vi "1A Helper - Init Sensor.vi"(8 "error in (no error)":errorcluster, 11 "VISA Refnum in":refnum<visa-resource-name>="COM1") -> (0 "error out":errorcluster, 3 "VISA Refnum out":refnum<visa-resource-name>)   [LabVIEW 2011]
doc: "This VI checks to see if the sensor is communicating on 4800 or 38400 baud and sets it to 38400 baud if it is not already."
uses:
  2-Think/2 Typedefs/indicator LED.ctl
  2-Think/2 Globals/2 Global.vi
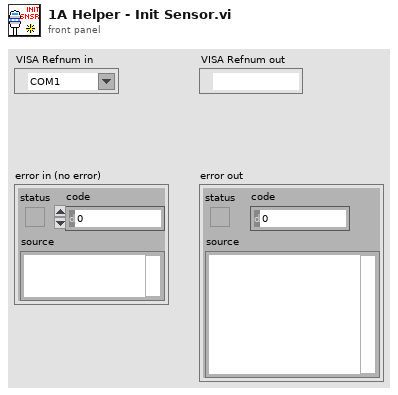
[diagram p1: front panel]
types:
  T1 = typedef "indicator LED.ctl" = bool
  T2 = typedef "generalized sensor status.ctl" = cluster{"Sensor Connected":T1, "Sensor Initialized":T1, "Sensor OK":T1, "Latest Error String":string, "GPS Lock":T1}
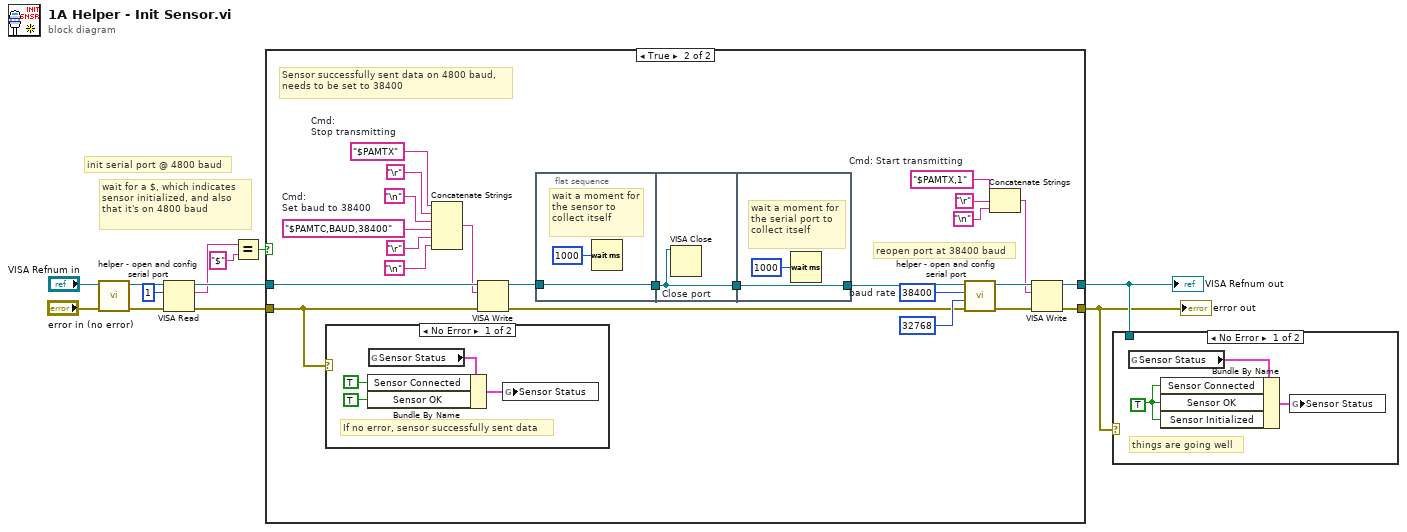
[diagram p0: block diagram]
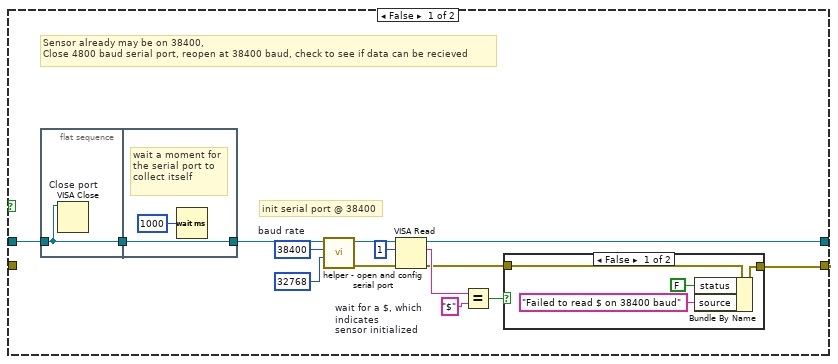
[diagram p2: hidden frame]
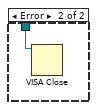
[diagram p5: hidden frame]
diagram:
  # "wait for a $, which indicates sensor initialized, and also that it's on 4800 baud"
  # "init serial port @ 4800 baud"
  n1 = call "helper - open and config serial port.vi"("error in (no error)"="error in (no error)", "VISA Refnum in"="VISA Refnum in") -> ("error out"=w6:errorcluster, "VISA Refnum out"=w7:refnum<visa-resource-name>)  [unwired: 8 in]
  n2 = VISA Read(VISA resource name=w7, byte count=u32 1, error in (no error)=w6) -> (VISA resource name out=w8:refnum<visa-resource-name>, read buffer=w2:string, error out=w5:errorcluster)  [unwired: 1 out]
  n3 = Equal? ("wait for a $, which indicates\nsensor initialized")(x=w2, y="$" ("x")) -> (x = y?=w4:bool)
  n4 = case shown="True" w4 {
    tunnel: [w19 w54] -> w10
    tunnel: w8 -> [w14 w46]
    tunnel: w5 -> [_ w35]
    tunnel: [w16 w41] -> w9
    frame False {
      w26 = u32 38400  # baud rate
      # "init serial port @ 38400"
      # "Sensor already may be on 38400,\nClose 4800 baud serial port, reopen at 38400 baud, check to see if data can be recieved"
      n5 = flat-sequence {
        tunnel: [w27] -> w15
        tunnel: w14 -> [w27]
        tunnel: [w29] -> w13
        tunnel: w15 -> [w29]
        frame #0 {
          n6 = VISA Close "Close port"(VISA resource name=w27) -> ()  [unwired: 1 in, 1 out]
        }
        frame #1 {
          # "wait a moment for the serial port to collect itself"
          n7 = Wait (ms)(milliseconds to wait=u32 1000) -> ()  [unwired: 1 out]
        }
      }
      n8 = call "helper - open and config serial port.vi"("Input\nbuffer size"=u32 32768 ("Input\nbuffer size"), "baud rate"=w26, "VISA Refnum in"=w13) -> ("error out"=w20:errorcluster, "VISA Refnum out"=w21:refnum<visa-resource-name>)  [unwired: 7 in]
      n9 = VISA Read(VISA resource name=w21, byte count=u32 1, error in (no error)=w20) -> (VISA resource name out=w19:refnum<visa-resource-name>, read buffer=w23:string, error out=w17:errorcluster)  [unwired: 1 out]
      n10 = Equal? "wait for a $, which indicates\nsensor initialized"(x=w23, y="$" ("x")) -> (x = y?=w18:bool)
      n11 = case shown="False" w18 {
        tunnel: w17 -> [w31 w34]
        tunnel: [w30 w34] -> w16
        frame False {
          n12 = Bundle By Name(cluster=w31, "status"=FALSE, "source"="Failed to read $ on 38400 baud") -> (w30:errorcluster)
        }
        frame True {
        }
      }
    }
    frame True {
      w40 = "$PAMTC,BAUD,38400"  # Cmd: Set baud to 38400
      w45 = "$PAMTX"  # Cmd: Stop transmitting
      w50 = "$PAMTX,1"  # Cmd: Start transmitting
      w56 = u32 38400  # baud rate
      # "Sensor successfully sent data on 4800 baud,\nneeds to be set to 38400"
      # "reopen port at 38400 baud"
      n13 = case shown="No Error" w35 {
        frame No Error {
          # "If no error, sensor successfully sent data"
          n14 = global read "2 Global.vi" "Sensor Status"() -> (w61:T2)
          n15 = Bundle By Name(cluster=w61, "Sensor Connected"=T1 TRUE, "Sensor OK"=T1 TRUE) -> (w62:T2)
          n16 = global write "2 Global.vi" "Sensor Status"(w62) -> ()
        }
        frame Error {
        }
      }
      n17 = Concatenate Strings(w45, "\r" ("Carriage Return Constant"), "\n", w40, "\r" ("Carriage Return Constant"), "\n") -> (w44:string)
      n18 = VISA Write(VISA resource name=w46, write buffer=w44, error in (no error)=w35) -> (VISA resource name out=w37:refnum<visa-resource-name>, error out=w36:errorcluster)  [unwired: 1 out]
      n19 = flat-sequence {
        tunnel: w37 -> [w63]
        tunnel: [w63] -> w58
        tunnel: w58 -> [w65]
        tunnel: [w65] -> w57
        tunnel: [w67] -> w55
        tunnel: w57 -> [w67]
        frame #0 {
          # "wait a moment for the sensor to collect itself"
          n20 = Wait (ms)(milliseconds to wait=u32 1000) -> ()  [unwired: 1 out]
        }
        frame #1 {
          n21 = VISA Close "Close port"(VISA resource name=w65) -> ()  [unwired: 1 in, 1 out]
        }
        frame #2 {
          # "wait a moment for the serial port to collect itself"
          n22 = Wait (ms)(milliseconds to wait=u32 1000) -> ()  [unwired: 1 out]
        }
      }
      n23 = call "helper - open and config serial port.vi"("error in (no error)"=w36, "Input\nbuffer size"=u32 32768 ("Input\nbuffer size"), "baud rate"=w56, "VISA Refnum in"=w55) -> ("error out"=w53:errorcluster, "VISA Refnum out"=w51:refnum<visa-resource-name>)  [unwired: 6 in]
      n24 = Concatenate Strings(w50, "\r" ("Carriage Return Constant"), "\n") -> (w47:string)
      n25 = VISA Write(VISA resource name=w51, write buffer=w47, error in (no error)=w53) -> (VISA resource name out=w54:refnum<visa-resource-name>, error out=w41:errorcluster)  [unwired: 1 out]
    }
  }
  "VISA Refnum out" <- w10
  "error out" <- w9
  n26 = case shown="No Error" w9 {
    tunnel: w10 -> [_ w71]
    frame No Error {
      w68 = T1 TRUE ("Sensor OK")
      # "things are going well"
      n27 = global read "2 Global.vi" "Sensor Status"() -> (w69:T2)
      n28 = Bundle By Name(cluster=w69, "Sensor Connected"=w68, "Sensor OK"=w68, "Sensor Initialized"=w68) -> (w70:T2)
      n29 = global write "2 Global.vi" "Sensor Status"(w70) -> ()
    }
    frame Error {
      n30 = VISA Close(VISA resource name=w71) -> ()  [unwired: 1 in, 1 out]
    }
  }
